vi "Unique File Name.vi"(8 "error in":errorcluster, 9 "Folder Name":string, 10 "APU Select":T1="<Select>", 11 "Crash Log?":bool) -> (0 "error out":errorcluster, 2 "Work Order Path":path, 3 "Unique File Path":path)   [LabVIEW 2018, in "File IO.lvlib"]
doc: "Create a unique file name and place in the Work Order folder."
uses:
  File IO.lvlib
  Controller (Host)/Public Controls/APU Select.ctl
  <vilib>/Utility/sysdir.llb/System Directory Type.ctl
  Controller (Host)/Controller (Host).lvlib
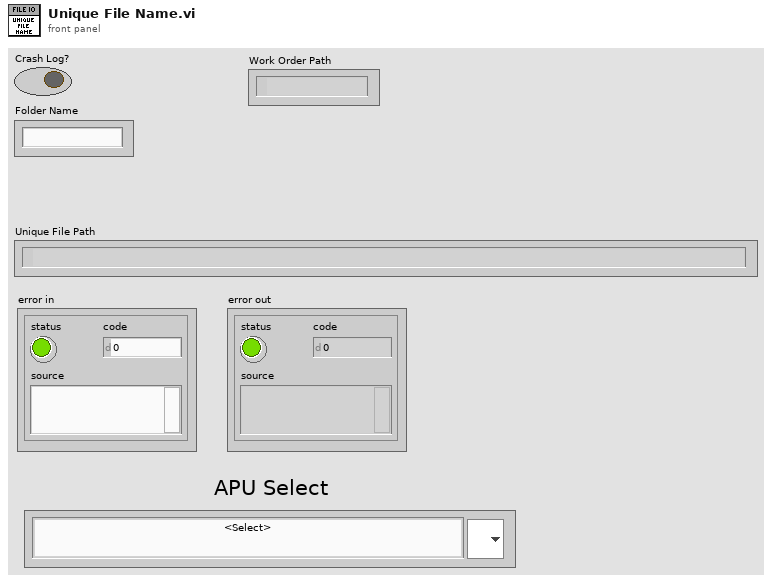
[diagram p1: front panel]
types:
  T1 = typedef "Controller (Host).lvlib/APU Select.ctl" = string
  T2 = typedef "System Directory Type.ctl" = i32
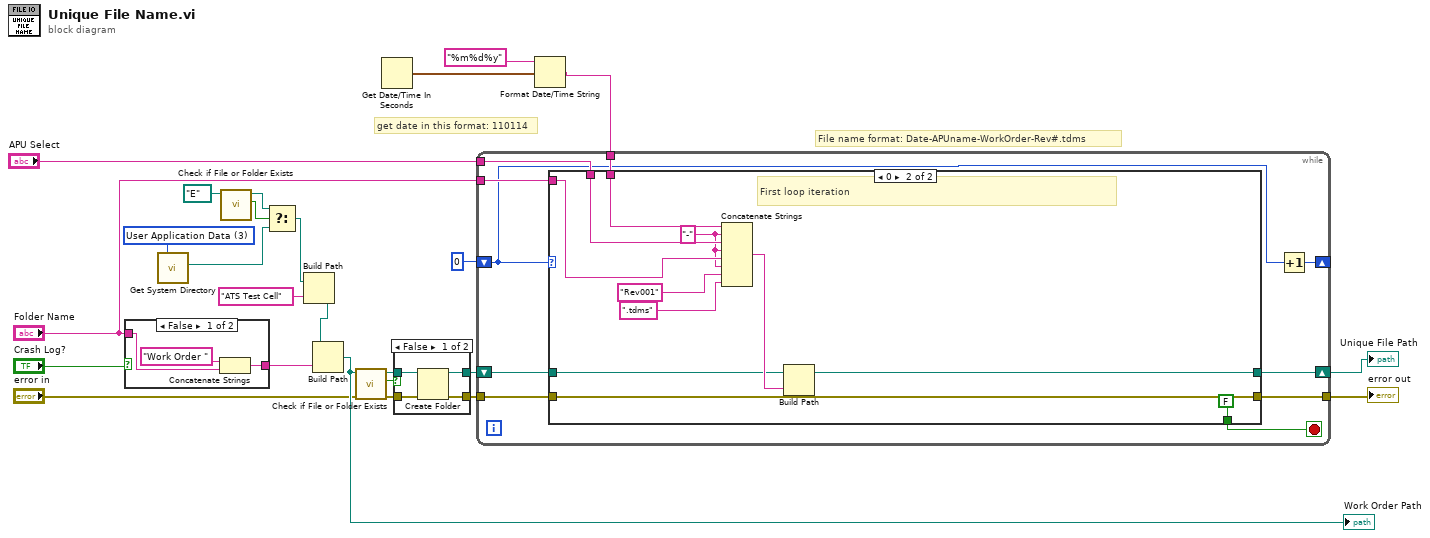
[diagram p0: block diagram]
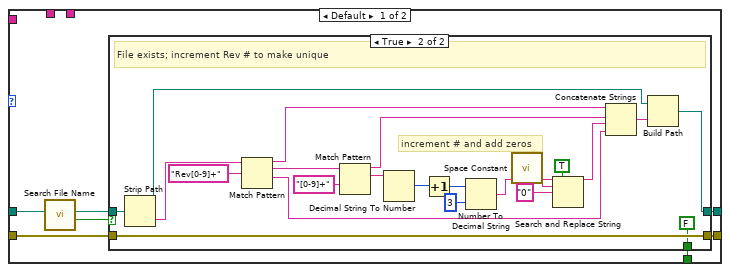
[diagram p4: hidden frame]
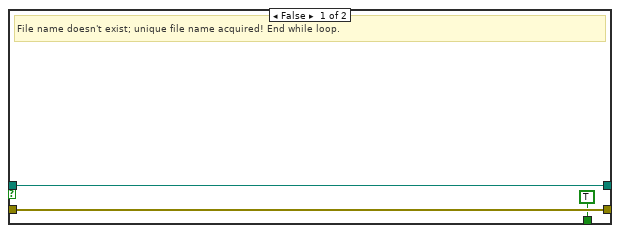
[diagram p5: hidden frame]
diagram:
  w20 = T2 3 items=["User Home"=0, "User Desktop"=1, "User Documents"=2, "User Application Data"=3, "User Preferences"=4, "User Temporary"=5, "Public Documents"=6, "Public Application Data"=7, "Public Preferences"=8, "Public Cache"=13, "System Core Libraries"=9, "System Installed Libraries"=10, "Application Files"=11, "Boot Volume Root"=12] ("system directory type")
  # "File name format: Date-APUname-WorkOrder-Rev#.tdms"
  # "get date in this format: 110114"
  n1 = case shown="False" "Crash Log?" {
    tunnel: [w27 w29] -> w15
    tunnel: "Folder Name" -> [w26 w29]
    frame False {
      n2 = Concatenate Strings("Work Order " ("string"), w26) -> (w27:string)
    }
    frame True {
      # "crash log"
    }
  }
  n3 = call <vilib>:"Get System Directory.vi"("system directory type"=w20) -> ("system directory"=w1:path)  [unwired: 10 in]
  n4 = call <vilib>:"Check if File or Folder Exists.vi"("path"=path "E:/") -> ("file or folder exists?"=w2:bool, "dup path"=w3:path)  [unwired: 8 in, 1 out]
  n5 = Select(t=w3, s=w2, f=w1) -> (s? t:f=w4:path)
  n6 = Build Path(base path=w4, name or relative path="ATS Test Cell") -> (appended path=w12:path)
  n7 = Build Path(base path=w12, name or relative path=w15) -> (appended path=w21:path)
  "Work Order Path" <- w21
  n8 = call <vilib>:"Check if File or Folder Exists.vi"("error in (no error)"="error in", "path"=w21) -> ("error out"=w24:errorcluster, "file or folder exists?"=w22:bool, "dup path"=w23:path)  [unwired: 7 in]
  n9 = Get Date/Time In Seconds() -> (seconds since 1Jan1904=w10:timestamp)
  n10 = case shown="False" w22 {
    tunnel: w23 -> [w33 w35]
    tunnel: [w32 w35] -> w17
    tunnel: w24 -> [w31 w34]
    tunnel: [w30 w34] -> w18
    frame False {
      n11 = Create Folder(path (use dialog)=w33, error in=w31) -> (created path=w32:path, error out=w30:errorcluster)  [unwired: 1 in, 1 out]
    }
    frame True {
    }
  }
  n12 = Format Date/Time String(time format string (%c)="%m%d%y", seconds (now)=w10) -> (date/time string=w9:string)  [unwired: 1 in]
  n13 = while {
    tunnel: w18 -> [w39]
    tunnel: [w45] -> w25
    tunnel: w9 -> [w44]
    tunnel: "APU Select" -> [w43]
    shift-right: [w42] -> w16
    shift-left: w17 -> [w40]
    tunnel: "Folder Name" -> [w38]
    shift-right: [w36] -> _
    shift-left: 0 -> [w37]
    stop <- w41 stop-if-true
    n14 = case shown="0" w37 {
      tunnel: w40 -> [w49 w86]
      tunnel: w39 -> [w48 w88]
      tunnel: [w52 w88] -> w45
      tunnel: w44 -> [_ w84]
      tunnel: w43 -> [_ w83]
      tunnel: [w51 w85] -> w42
      tunnel: [w50 FALSE] -> w41
      tunnel: w38 -> [_ w82]
      frame Default {
        n15 = call "Search File Name.vi"("File Path In"=w49) -> ("File name found?"=w46:bool, "File Path Out"=w47:path)  [unwired: 9 in]
        n16 = case shown="True" w46 {
          tunnel: w48 -> [w55 w77]
          tunnel: [w55 w77] -> w52
          tunnel: [w53 w75] -> w51
          tunnel: [TRUE FALSE] -> w50
          tunnel: w47 -> [w53 w66]
          frame False {
            # "File name doesn't exist; unique file name acquired! End while loop."
          }
          frame True {
            # "increment # and add zeros"
            # "File exists; increment Rev # to make unique"
            n17 = Strip Path(path=w66) -> (stripped path=w65:path, name=w73:string)
            n18 = Match Pattern(string=w73, regular expression="Rev[0-9]+") -> (before substring=w64:string, match substring=w72:string, after substring=w56:string)  [unwired: 1 in, 1 out]
            n19 = Match Pattern(string=w72, regular expression="[0-9]+") -> (before substring=w63:string, match substring=w68:string)  [unwired: 1 in, 2 out]
            n20 = Decimal String To Number(string=w68) -> (number=w70:i32)  [unwired: 2 in, 1 out]
            n21 = Increment(x=w70) -> (x+1=w62:i32)
            n22 = Number To Decimal String(number=w62, width (-)=i16 3) -> (decimal integer string=w60:string)
            n23 = call <vilib>:"Space Constant.vi"() -> ("String"=w59:string)
            n24 = Search and Replace String(replace all?=TRUE ("replace all? (F)"), input string=w60, search string=w59, replace string="0" ("replace string (\"\")")) -> (result string=w67:string)  [unwired: 4 in, 3 out]
            n25 = Concatenate Strings(w64, w63, w67, w56) -> (w76:string)
            n26 = Build Path(base path=w65, name or relative path=w76) -> (appended path=w75:path)
          }
        }
      }
      frame 0 {
        w78 = "-" ("string")
        # "First loop iteration"
        n27 = Concatenate Strings(w84, w78, w83, w78, w82, w78, "Rev001" ("string"), ".tdms" ("string")) -> (w87:string)
        n28 = Build Path(base path=w86, name or relative path=w87) -> (appended path=w85:path)
      }
    }
    n29 = Increment(x=w37) -> (x+1=w36:i32)
  }
  "error out" <- w25
  "Unique File Path" <- w16
